vi "Update Test Timer.vi"(8 "error in (no error)":errorcluster, 10 "Timeout Value":i32=1000, 11 "Timing Engine Tester in":refnum<class "Timing Engine Tester.lvclass">) -> (0 "error out":errorcluster, 3 "Timing Engine Tester out":refnum<class "Timing Engine Tester.lvclass">)   [LabVIEW 2016, in "Assert API Components.lvlib" / "Assert Display.lvlib" / "Timing Engine Tester.lvlib" / "Timing Engine Tester.lvclass"]
uses:
  Timing Engine Tester.lvclass
  Timing Engine Tester.lvclass/Timing Engine Tester.ctl
  Core/Timing Engine/Timing Engine Messages/Timer Update Msg/Timer Update Msg.lvclass/Timer Update Msg.ctl
  <vilib>/ActorFramework/Message Enqueuer/Message Enqueuer.lvclass/Message Enqueuer.ctl
  <vilib>/ActorFramework/Message Enqueuer/Enqueue.vi
  Core/Timing Engine/Timing Engine Messages/Timer Update Msg/Timer Update Msg.lvclass
  C:/Program Files (x86)/National Instruments/LabVIEW 2016/vi.lib/ActorFramework/Message/Message.lvclass
  <vilib>/Utility/LVClass/Get LV Class Name.vi
  <resource>/AFDebug/Generate Trace for Message.vi
  <vilib>/ActorFramework/Message Priority Queue/Priority Enqueue.vi
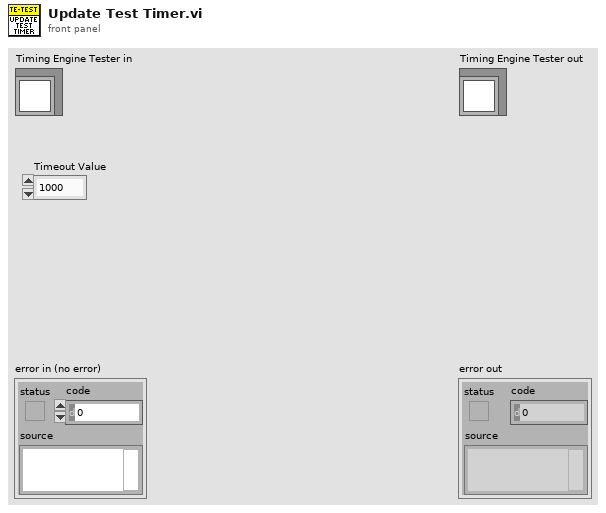
[diagram p1: front panel]
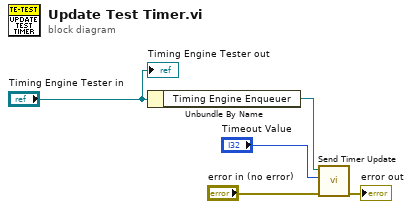
[diagram p0: block diagram]
diagram:
  n1 = Unbundle By Name("Timing Engine Tester in") -> ("Timing Engine Enqueuer"=w4:refnum<class "Message Enqueuer.lvclass">)
  n2 = call "Send Timer Update.vi"("error in (no error)"="error in (no error)", "Timeout Value"="Timeout Value", "Message Enqueuer"=w4) -> ("error out"=→"error out":errorcluster)  [unwired: 7 in, 1 out]
  "Timing Engine Tester out" <- "Timing Engine Tester in"
